vi "Cluster Non-profile values.vi"(8 "error in (no error)":errorcluster) -> (0 "error out":errorcluster, 3 "Non-profile parameters cluster":T1)   [LabVIEW 2017]
uses:
  User Interface/User profiles code/Typedefs/Non-profile parameters cluster.ctl
  Typedefs/HW config states enum.ctl
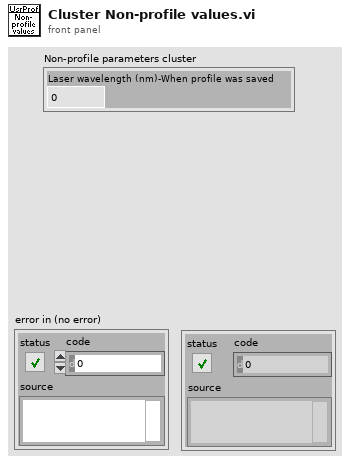
[diagram p1: front panel]
types:
  T1 = typedef "Non-profile parameters cluster.ctl" = cluster{"Laser wavelength (nm)-When profile was saved":dbl}
  T2 = typedef "HW config states enum.ctl" = enum16{"Load from file", "Save to file", "Write all", "Read all", "Write XY stage settings", "Write DAQ FPGA settings", "Write Control FPGA settings", "Write Phys Channels", "Clear", "Compare from file"}
  T3 = typedef "System Configuration.ctl" = cluster{"Laser wavelength (nm)":dbl, "DAQ FPGA System":T4, "Control system":T6}
  T4 = typedef "DAQ FPGA system config.ctl" = cluster{"Clock Freq (MHz) ":dbl, "Samples Wait after Trigger":u16, "AOD fill":u16, "StartupDelay":i32, "Slip Cycle (clock cycles)":u32, "Add Cycle":bool, "Ref":T5}
  T5 = typedef "FPGA Ref.ctl" = refnum<k20>
  T6 = typedef "CTRL system config.ctl" = cluster{"AOD 1 Amplitude":i16, "AOD 2 Amplitude":i16, "AOD 3 Amplitude":i16, "AOD 4 Amplitude":i16, "AOD 5 Amplitude":i16, "AOD 6 Amplitude":i16, "T0 (ns)":dbl, "Ta (ns)":dbl, "Data Time Interval (ns)":dbl, "Ctrl FPGA Clock (MHz)":dbl, "Ethernet opened":bool}
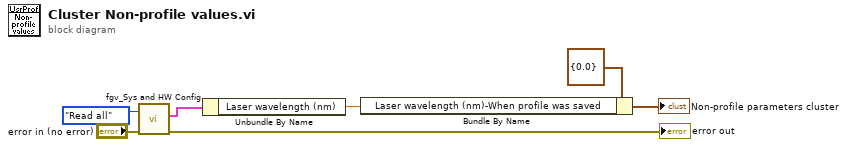
[diagram p0: block diagram]
diagram:
  n1 = call "fgv_Sys and HW Config.vi"("Function"=HW_config_states_enum."Read all", "error in (no error)"="error in (no error)") -> ("error out"=→"error out":errorcluster, "System Config OUT"=w1:T3)  [unwired: 7 in, 1 out]
  n2 = Unbundle By Name(w1) -> ("Laser wavelength (nm)"=w7:dbl)
  n3 = Bundle By Name(cluster=T1 {"Laser wavelength (nm)-When profile was saved"=0.0} ("Non-profile parameters cluster"), "Laser wavelength (nm)-When profile was saved"=w7) -> (→"Non-profile parameters cluster":T1)
